vi "BMU参数读取-Auto.vi"(7 "Socket":dbl, 8 "CAN端口":u16(ring), 9 "设备索引号":u16(ring), 10 "CAN卡类型":u32(ring)=21, 11 "从板号":u8=1) -> (3 "成功?":bool)   [LabVIEW 2013] (continued)
      n13 = property on="电池额定容量(A)" class="DigNum (严格)"("Disabled"=w44) -> ()  [unwired: 2 in, 2 out]
      n14 = local write "主从选择"(enum32{"主板", "从板"}."从板" ("主从选择")) -> ()
      n15 = property on="SOC(%)" class="DigNum (严格)"("Disabled"=w44) -> ()  [unwired: 2 in, 2 out]
      n16 = local write "等级 2"(T20."从板信息" ("等级 2")) -> ()
      n17 = local write "主板2"(T9."项目信息" ("主从板")) -> ()
      n18 = property class="MCListbox (严格)"(reference=w49, "ItemNames"=w45) -> ()  [unwired: 1 in, 2 out]
      n19 = property class="MCListbox (严格)"(reference=w48, "ItemNames"=w45) -> ()  [unwired: 1 in, 2 out]
      n20 = property class="MCListbox (严格)"(reference=w47, "ItemNames"=w45) -> ()  [unwired: 1 in, 2 out]
      n21 = property class="Bool (严格)"(reference=w66, "BoolText.TextColor"=u32 87470) -> ()  [unwired: 1 in, 2 out]
      n22 = property class="Bool (严格)"(reference=w67, "BoolText.TextColor"=w41) -> ()  [unwired: 1 in, 2 out]
      n23 = property on="从板号" class="DigNum (严格)"("Visible"=TRUE ("可见")) -> ()  [unwired: 2 in, 2 out]
      n24 = local write "主从板"(enum32{"单选选项2", "单选选项1"}."单选选项1" ("主从板")) -> ()
      n25 = property on="项目信息2" class="Clust (严格)"("DisabledEnum"=w44) -> ()  [unwired: 2 in, 2 out]
      n26 = property on="系统时钟" class="Str"("Disabled"=w44) -> ()  [unwired: 2 in, 2 out]
      n27 = property on="配置文件版本" class="Str"("Disabled"=w44) -> ()  [unwired: 2 in, 2 out]
      n28 = property on="车架(牌)号" class="Str"("Disabled"=w44) -> ()  [unwired: 2 in, 2 out]
      n29 = property on="产品编号" class="Str"("Disabled"=w44) -> ()  [unwired: 2 in, 2 out]
      n30 = property on="单选选项2 2" class="Bool (严格)"("BoolText.TextColor"=w41) -> ()  [unwired: 2 in, 2 out]
      n31 = property on="单选选项2" class="Bool (严格)"("BoolText.TextColor"=w41) -> ()  [unwired: 2 in, 2 out]
      n32 = property on="单选选项1" class="Bool (严格)"("BoolText.TextColor"=u32 5898201) -> ()  [unwired: 2 in, 2 out]
      n33 = property on="从板号" class="DigNum (严格)"("NumText.BGColor"=w41) -> ()  [unwired: 2 in, 2 out]
      n34 = local write "面板选择"(T7."读写参数" ("面板选择")) -> ()
      n35 = local write "主界面选项"(enum32{"单选选项1", "单选选项2", "单选选项2 2", "单选选项2 3"}."单选选项1" ("主界面选项")) -> ()
      n36 = local write "判定3"(w51) -> ()
      n37 = local write "清BUFF"(w51) -> ()
      n38 = local write "1"(w51) -> ()
      n39 = property on="从板个数" class="DigNum (严格)"("Visible"=w51) -> ()  [unwired: 2 in, 2 out]
      n40 = property on="从板个数" class="DigNum (严格)"("NumText.BGColor"=u32 16448250) -> ()  [unwired: 2 in, 2 out]
      n41 = Not(x=w51) -> (.not. x?=w70:bool)
      n42 = property on="主板选项" class="Tree (严格)"("Visible"=w51) -> ()  [unwired: 2 in, 2 out]
      n43 = property on="全部写入" class="Bool (严格)"("DisabledEnum"=2) -> ()  [unwired: 2 in, 2 out]
      n44 = property on="当前从板板号" class="DigNum (严格)"("Visible"=w70) -> ()  [unwired: 2 in, 2 out]
      n45 = property on="从板选项" class="Tree (严格)"("Visible"=w70) -> ()  [unwired: 2 in, 2 out]
      n46 = control-ref of="结果"() -> (w57:refnum<vi>)
      n47 = control-ref of="结果"() -> (w54:refnum<vi>)
      n48 = local write "强制停止版本读取"(w43) -> ()
      n49 = local write "强制终止读写标记"(w43) -> ()
      n50 = control-ref of="项目信息"() -> (w55:refnum<vi>)
      n51 = local write "判定2"(w43) -> ()
      n52 = local write "停止"(w43) -> ()
      n53 = local write "控制1"(w43) -> ()
      n54 = local write "消除"(w43) -> ()
      n55 = global write "EV05全局变量1.vi" "授权功能"(w43) -> ()
      n56 = local write "继电器超时处理"(w43) -> ()
      n57 = local write "1 6"(w43) -> ()
      n58 = local write "1 7"(w43) -> ()
      n59 = local write "1 8"(w43) -> ()
      n60 = local write "1 9"(w43) -> ()
      n61 = local write "1 10"(w43) -> ()
      n62 = local write "1 2"(w43) -> ()
      n63 = local write "1 3"(w43) -> ()
      n64 = local write "1 4"(w43) -> ()
      n65 = local write "1 5"(w43) -> ()
      n66 = local write "1 11"(w43) -> ()
      n67 = for {
        N: 100 -> [_]
        tunnel: w57 -> [w98]
        i -> [w96]
        n68 = Bundle(w96, 0) -> (w94:cluster{i32, i32})  [unwired: 1 out]
        n69 = property class="MCListbox (严格)"(reference=w98, "ActiveCell"=w94, "CellBG"=u32 16448250) -> ()  [unwired: 1 in, 2 out]
      }
      n70 = for {
        N: 100 -> [_]
        tunnel: w55 -> [w93]
        i -> [w92]
        n71 = Bundle(w92, 0) -> (w90:cluster{i32, i32})  [unwired: 1 out]
        n72 = property class="Tbl (严格)"(reference=w93, "Active Cell"=w90, "Cell BG Color"=u32 16448250) -> ()  [unwired: 1 in, 2 out]
      }
      n73 = for {
        N: 100 -> [_]
        tunnel: w54 -> [w103]
        i -> [w101]
        n74 = Bundle(w101, 0) -> (w99:cluster{i32, i32})  [unwired: 1 out]
        n75 = property class="MCListbox (严格)"(reference=w103, "ActiveCell"=w99, "CellBG"=u32 16448250) -> ()  [unwired: 1 in, 2 out]
      }
      n76 = disable-structure shown="禁用" {
        disable-tunnel: [w71 _] -> w50
        frame Disabled {
          n77 = stacked-sequence {
            tunnel: [_ _ w77] -> w71
            frame #0 {
              w72 = u32 4 items=["PCI5121"=1, "PCI9810"=2, "USBCAN1"=3, "USBCAN2"=4, "PCI9820"=5, "PCI5110"=7, "CANLite(mini)"=8, "ISA9620"=9, "ISA5420"=10, "PC104CAN"=11, "DNP9810"=13, "PCI9840B"=14, "PC104C2"=15, "PCI9820I"=16, "pec9920"=18, "USBCAN_E_U"=20, "USBCAN_2E_U"=21] ("CAN卡类型")
              n78 = local write "CAN卡类型"(w72) -> ()
            }
            frame #1 {
              n79 = local read "设备索引号"() -> (w74:u16)
              n80 = local read "CAN卡类型"() -> (w73:u32)
              n81 = local read "CAN端口"() -> (w75:u16)
              n82 = dll-call lib="PTH1abs FBluewave New EnergySVN_WorkAutoTest_TestStandtrunkAutoTest_TestStandDriverZlgCanBHN01è¯»ååæ°data\nkerneldlls\nusbcan.dll" fn="VCI_ClearBuffer"("DeviceType"=w73, "DeviceInd"=w74, "CANInd"=w75) -> (error out=w76:errorcluster)  [unwired: 4 in, 4 out]
              n83 = call <vilib>:"Clear Errors.vi"("error in (no error)"=w76) -> ()  [unwired: 6 in, 1 out]
            }
            frame #2 {
              w84 = u8 0 items=["Normal", "Listen Only"] ("工作方式")
              w83 = u8 1 items=["Dual Filter", "Single Filter"] ("滤波方式")
              n84 = local read "CAN卡类型"() -> (w78:u32)
              n85 = local read "设备索引号"() -> (w79:u16)
              n86 = local read "CAN端口"() -> (w80:u16)
              n87 = call "CAN_Init-8.6.vi"("CAN卡类型"=w78, "设备索引号"=w79, "CAN端口"=w80, "操作类型"=enum16{"初始化CAN", "关闭CAN"}."初始化CAN", "滤波方式"=w83, "Accept Code"=u32 3221225472, "簇"=T22 {"打开CAN"=TRUE, "初始化CAN"=TRUE, "开始CAN"=TRUE, "重启"=FALSE, "关闭CAN"=FALSE}, "Mask Code"=u32 1073741823 ("Accept Code"), "工作方式"=w84, "是否滤波"=TRUE, "滤波选择"=T21 {"fiter_mode"=1, "fiter_endid"=402653184, "fiter_startid"=419430399}) -> ("error out"=w77:errorcluster)  [unwired: 3 in, 5 out]
            }
          }
        }
        frame Enabled {
        }
      }
      n88 = local write "加热继电器(从)"(w43) -> ()
      n89 = local write "风机继电器(从)"(w43) -> ()
      n90 = local write "DO1"(w43) -> ()
      n91 = local write "DO2"(w43) -> ()
      n92 = local write "DO1 2"(w43) -> ()
      n93 = local write "正级继电器"(w43) -> ()
      n94 = local write "负级继电器"(w43) -> ()
      n95 = local write "加热继电器"(w43) -> ()
      n96 = local write "充电继电器"(w43) -> ()
      n97 = local write "风机继电器"(w43) -> ()
      n98 = local write "预充电继电器"(w43) -> ()
      n99 = property on="保存版本信息" class="Bool (严格)"("Visible"=w43) -> ()  [unwired: 2 in, 2 out]
      n100 = property on="单个读取" class="Bool (严格)"("Visible"=w43) -> ()  [unwired: 2 in, 2 out]
      n101 = property on="单个写入" class="Bool (严格)"("Visible"=w43) -> ()  [unwired: 2 in, 2 out]
      n102 = local write "正级继电器 12"(w43) -> ()
      n103 = local write "正级继电器 2"(w43) -> ()
      n104 = local write "正级继电器 3"(w43) -> ()
      n105 = local write "正级继电器 4"(w43) -> ()
      n106 = local write "正级继电器 5"(w43) -> ()
      n107 = local write "正级继电器 6"(w43) -> ()
      n108 = local write "正级继电器 7"(w43) -> ()
      n109 = local write "正级继电器 8"(w43) -> ()
      n110 = local write "正级继电器 9"(w43) -> ()
      n111 = local write "正级继电器 10"(w43) -> ()
      n112 = local write "正级继电器 11"(w43) -> ()
      "电池故障" <- w45
      "模块版本值" <- w62
      "硬件版本" <- w63
      "模块版本名称" <- w62
      "平台软件版本" <- w63
      "项目软件版本" <- w63
      "模块个数" <- u8[] [0, 0, 0, 0, 0, 0, 0, 0, 0, 0, 0, 0, 0, 0, 0, 0, 0, 0, 0, 0, 0, 0, 0, 0, 0, 0, 0, 0, 0, 0, 0, 0] ("模块个数")
    }
  }
  n113 = stacked-sequence {
    tunnel: [w104] -> w29
    frame #0 {
      n114 = call <vilib>:"Set Busy.vi"() -> ()  [unwired: 10 in, 2 out]
      n115 = disable-structure shown="禁用" {
        frame Disabled {
          n116 = control-ref of="主板选项"() -> (w223:refnum<vi>)
          n117 = stacked-sequence {
            tunnel: w223 -> [w225 w383 w421]
            frame #0 {
              # "加热和充电控制参数"
              n118 = global read "功能码全局.vi" "主板控制类信息10"() -> (w235:bool[])
              n119 = Index Array(array=w235) -> (element #5=w229:bool, element #6=w227:bool, element #7=w228:bool, element #8=w226:bool)  [unwired: 8 in, 4 out]
              n120 = Not Or(1:w228, 2:w229) -> (0:w234:bool)
              n121 = Not Or(1:w226, 2:w227) -> (0:w232:bool)
              n122 = for {
                N: 8 -> [_]
                tunnel: w225 -> [w355]
                tunnel: w234 -> [w351]
                tunnel: [w350] -> w233
                i -> [w353]
                n123 = Add(x=w353, y=69) -> (x+y=w354:i32)
                n124 = property class="Tree (严格)"(reference=w355, "Active Item Row Number"=w354, "Disabled?"=w351) -> (error out=w350:errorcluster)  [unwired: 1 in, 1 out]
              }
              n125 = for {
                N: 9 -> [_]
                tunnel: w225 -> [w349]
                tunnel: w232 -> [w345]
                tunnel: w233 -> [w344]
                tunnel: [w343] -> w224
                i -> [w347]
                n126 = Add(x=w347, y=77) -> (x+y=w348:i32)
                n127 = property class="Tree (严格)"(reference=w349, error in=w344, "Active Item Row Number"=w348, "Disabled?"=w345) -> (error out=w343:errorcluster)  [unwired: 1 out]
              }
              n128 = stacked-sequence {
                tunnel: w225 -> [w255 _ _]
                tunnel: w224 -> [w254 _ _]
                frame #0 {
                  # "电池信息"
                  n129 = global read "功能码全局.vi" "主板版本号11"() -> (w256:bool[])
                  n130 = global read "功能码全局.vi" "主板项目信息4"() -> (w238:bool[])
                  n131 = Index Array(array=w256) -> (element #1=w252:bool, element #2=w251:bool, element #3=w245:bool, element #4=w239:bool, element #6=w244:bool, element #7=w243:bool, element #8=w242:bool)  [unwired: 8 in, 1 out]
                  n132 = Index Array(array=w238, index=4 ("索引")) -> (element=w236:bool)
                  n133 = Or(x=w245, y=w239) -> (x .or. y?=w240:bool)
                  n134 = Not(x=w243) -> (.not. x?=w247:bool)
                  n135 = Not(x=w242) -> (.not. x?=w246:bool)
                  n136 = Not(x=w244) -> (.not. x?=w248:bool)
                  n137 = property on="硬件版本号" class="Str"("Visible"=w245) -> ()  [unwired: 2 in, 2 out]
                  n138 = property on="读硬件版本号" class="Bool (严格)"("Visible"=w245) -> ()  [unwired: 2 in, 2 out]
                  n139 = property on="项目软件版本号" class="Str"("Visible"=w245) -> ()  [unwired: 2 in, 2 out]
                  n140 = property on="项目软本读取" class="Bool (严格)"("Visible"=w245) -> ()  [unwired: 2 in, 2 out]
                  n141 = property on="继电器屏1 2" class="TabCtl (严格)"("Visible"=w248) -> ()  [unwired: 2 in, 2 out]
                  n142 = property on="均衡屏" class="TabCtl (严格)"("Visible"=w246) -> ()  [unwired: 2 in, 2 out]
                  n143 = property on="继电器屏1 2" class="TabCtl (严格)"("Visible"=w248) -> ()  [unwired: 2 in, 2 out]
                  n144 = property on="DO屏" class="TabCtl (严格)"("Visible"=w247) -> ()  [unwired: 2 in, 2 out]
                  n145 = Compound Arithmetic op=OR(w244, w243, w242) -> (w241:bool)
                  n146 = Not Or(1:w251, 2:w252) -> (0:w250:bool)
                  n147 = stacked-sequence {
                    tunnel: w241 -> [_ w261 _]
                    tunnel: w240 -> [_ _ w265]
                    tunnel: w236 -> [w257 _ _]
                    frame #0 {
                      n148 = case shown="真" w257 {
                        frame False {
                        }
                        frame True {
                          n149 = local write "主界面选项"(enum32{"单选选项1", "单选选项2", "单选选项2 2", "单选选项2 3"}."单选选项2 3" ("主界面选项")) -> ()
                          n150 = local write "面板选择"(T7."高压板校正" ("面板选择")) -> ()
                        }
                      }
                      n151 = control-ref of="单选选项2 3"() -> (w258:refnum<vi>)
                      n152 = property class="Bool (严格)"(reference=w258, "Visible"=w257) -> ()  [unwired: 1 in, 2 out]
                    }
                    frame #1 {
                      n153 = control-ref of="单选选项2 2"() -> (w262:refnum<vi>)
                      n154 = case shown="真" w261 {
                        frame False {
                        }
                        frame True {
                          n155 = local write "主界面选项"(enum32{"单选选项1", "单选选项2", "单选选项2 2", "单选选项2 3"}."单选选项2 2" ("主界面选项")) -> ()
                          n156 = local write "面板选择"(enum32{"读写参数", "版本读取", "其它诊断"}."其它诊断" ("选项卡控件 2")) -> ()
                        }
                      }
                      n157 = property class="Bool (严格)"(reference=w262, "Visible"=w261) -> ()  [unwired: 1 in, 2 out]
                    }
                    frame #2 {
                      n158 = control-ref of="单选选项2"() -> (w266:refnum<vi>)
                      n159 = case shown="真" w265 {
                        frame False {
                        }
                        frame True {
                          n160 = local write "主界面选项"(enum32{"单选选项1", "单选选项2", "单选选项2 2", "单选选项2 3"}."单选选项2" ("主界面选项")) -> ()
                          n161 = local write "面板选择"(enum32{"读写参数", "版本读取", "其它诊断"}."版本读取" ("选项卡控件 2")) -> ()
                        }
                      }
                      n162 = property class="Bool (严格)"(reference=w266, "Visible"=w265) -> ()  [unwired: 1 in, 2 out]
                    }
                  }
                  n163 = for {
                    N: 5 -> [_]
                    tunnel: w255 -> [w275]
                    tunnel: w250 -> [w271]
                    tunnel: w254 -> [w270]
                    tunnel: [w269] -> w253
                    i -> [w273]
                    n164 = Add(x=w273, y=86) -> (x+y=w274:i32)
                    n165 = property class="Tree (严格)"(reference=w275, error in=w270, "Active Item Row Number"=w274, "Disabled?"=w271) -> (error out=w269:errorcluster)  [unwired: 1 out]
                  }
                  n166 = property on="模块软件版本 2" class="MCListbox (严格)"("Visible"=w239) -> ()  [unwired: 2 in, 2 out]
                  n167 = property on="模块软件版本" class="Enum (严格)"("Visible"=w239) -> ()  [unwired: 2 in, 2 out]
                  n168 = property on="平台软件版本号" class="Str"("Visible"=w239) -> ()  [unwired: 2 in, 2 out]
                  n169 = property on="模块版本读取" class="Bool (严格)"("Visible"=w239) -> ()  [unwired: 2 in, 2 out]
                  n170 = property on="平台软件版本读取" class="Bool (严格)"("Visible"=w239) -> ()  [unwired: 2 in, 2 out]
                  n171 = call <vilib>:"Clear Errors.vi"("error in (no error)"=w253) -> ()  [unwired: 6 in, 1 out]
                }
                frame #1 {
                  n172 = global read "功能码全局.vi" "主板项目信息7"() -> (w315:bool[])
                  n173 = global read "功能码全局.vi" "主板控制类信息10"() -> (w311:bool[])
                  n174 = global read "功能码全局.vi" "主板故障阀值9"() -> (w314:bool[])
                  n175 = global read "功能码全局.vi" "主板项目信息4"() -> (w293:bool[])
                  n176 = global read "功能码全局.vi" "主板项目信息5"() -> (w302:bool[])
                  n177 = global read "功能码全局.vi" "主板项目信息6"() -> (w292:bool[])
                  n178 = global read "功能码全局.vi" "主板版本号11"() -> (w301:bool[])
                  n179 = Delete From Array(array=w292, length=1 ("长度"), index=0 ("索引")) -> (deleted portion=w303:bool[], array with subset deleted=w319:bool[])
                  n180 = Index Array(array=w293, index #1=5 ("索引"), index #2=6 ("索引"), index #3=7 ("索引")) -> (element #1=w304:bool, element #2=w320:bool, element #3=w276:bool)
                  n181 = Index Array(array=w301) -> (element #1=w308:bool, element #2=w324:bool)  [unwired: 2 in]
                  n182 = Array Subset(array=w314, index=2 ("索引"), length=3 ("长度")) -> (w306:bool[])
                  n183 = Delete From Array(array=w315, length=3 ("索引"), index=2 ("长度")) -> (deleted portion=w305:bool[], array with subset deleted=w321:bool[])
                  n184 = Array Subset(array=w311, index=4 ("索引"), length=2 ("长度")) -> (w307:bool[])
                  n185 = global read "功能码全局.vi" "18"() -> (w284:bool[])
                  n186 = global read "功能码全局.vi" "16"() -> (w285:bool[])
                  n187 = Insert Into Array(array=w302, new element #1=w303, new element #2=w304, new element #3=w305, new element #4=w306, new element #5=w307, new element #6=w308) -> (w325:bool[])  [unwired: 1 in]
                  n188 = Array Subset(array=w311, index=6 ("索引"), length=2 ("长度")) -> (w323:bool[])
                  n189 = Array Subset(array=w314, index=5 ("索引"), length=3 ("长度")) -> (w322:bool[])
                  n190 = And Array Elements(Boolean array=w325) -> (logical AND=w290:bool)
                  n191 = Array Subset(array=w284, index=0 ("索引"), length=8 ("长度")) -> (w282:bool[])
                  n192 = Array Subset(array=w285, index=4 ("索引"), length=4 ("长度")) -> (w281:bool[])
                  n193 = Or Array Elements(Boolean array=w325) -> (logical OR=w277:bool)
                  n194 = Insert Into Array(array=w319, new element #1=w320, new element #2=w321, new element #3=w322, new element #4=w323, new element #5=w324) -> (w326:bool[])  [unwired: 1 in]
                  n195 = property on="全部读取" class="Bool (严格)"("Visible"=w290) -> ()  [unwired: 2 in, 2 out]
                  n196 = global read "功能码全局.vi" "15"() -> (w283:bool[])
                  n197 = And Array Elements(Boolean array=w326) -> (logical AND=w291:bool)
                  n198 = property on="全部写入" class="Bool (严格)"("Visible"=w291) -> ()  [unwired: 2 in, 2 out]
                  n199 = Or Array Elements(Boolean array=w326) -> (logical OR=w327:bool)
                  n200 = Insert Into Array(array=w283, new element #1=w282, new element #2=w281) -> (w280:bool[])  [unwired: 1 in]
                  n201 = Or Array Elements(Boolean array=w280) -> (logical OR=w279:bool)
                  n202 = Compound Arithmetic op=OR(w276, w277, w327, w279) -> (w328:bool)
                  n203 = case shown="真" w328 {
                    frame False {
                    }
                    frame True {
                      n204 = local write "主界面选项"(enum32{"单选选项1", "单选选项2", "单选选项2 2", "单选选项2 3"}."单选选项1" ("主界面选项")) -> ()
                      n205 = local write "面板选择"(enum32{"读写参数", "版本读取", "其它诊断"}."读写参数" ("选项卡控件 2")) -> ()
                    }
                  }
                  n206 = property on="单选选项1" class="Bool (严格)"("Visible"=w328) -> ()  [unwired: 2 in, 2 out]
                }
                frame #2 {
                  n207 = control-ref of="单选选项2 2"() -> (w335:refnum<vi>)
                  n208 = control-ref of="单选选项2 3"() -> (w331:refnum<vi>)
                  n209 = control-ref of="单选选项2"() -> (w337:refnum<vi>)
                  n210 = control-ref of="单选选项1"() -> (w336:refnum<vi>)
                  n211 = local read "主界面选项"() -> (w340:enum32{"单选选项1", "单选选项2", "单选选项2 2", "单选选项2 3"})
                  n212 = Build Array(w336, w337, w335, w331) -> (w334:refnum<vi>[])
                  n213 = Delete From Array(array=w334, index=w340) -> (deleted portion=w338:refnum<vi>, array with subset deleted=w339:refnum<vi>[])  [unwired: 1 in]
                  n214 = property class="Bool (严格)"(reference=w338, "BoolText.TextColor"=u32 87470) -> ()  [unwired: 1 in, 2 out]
                  n215 = for {
                    tunnel: u32 16777215 -> [w342]
                    tunnel: w339 -> [w341] mode=indexing
                    n216 = property class="Bool (严格)"(reference=w341, "BoolText.TextColor"=w342) -> ()  [unwired: 1 in, 2 out]
                  }
                }
              }
            }
            frame #1 {
              # "项目信息"
              # "SOC"
              # "SOH"
              # "电池额定实际容量"
              # "车牌号"
              # "产品编号"
              # "电压个数"
              # "通道电压数"
              # "温度个数"
              # "电压起始值"
              # "温度起始值"
              # "配置文件版本"
              # "系统时钟"
              # "校正时钟"
              n217 = global read "功能码全局.vi" "主板项目信息5"() -> (w416:bool[])
              n218 = global read "功能码全局.vi" "主板项目信息6"() -> (w415:bool[])
              n219 = global read "功能码全局.vi" "主板项目信息7"() -> (w392:bool[])
              n220 = global read "功能码全局.vi" "主板项目信息4"() -> (w363:bool[])
              n221 = Index Array(array=w416) -> (element #1=w413:bool, element #2=w410:bool, element #3=w407:bool, element #4=w404:bool, element #5=w400:bool, element #6=w398:bool, element #7=w395:bool, element #8=w391:bool)  [unwired: 8 in]
              n222 = Index Array(array=w415) -> (element #1=w388:bool, element #2=w412:bool, element #3=w409:bool, element #4=w406:bool, element #5=w403:bool, element #6=w399:bool, element #7=w397:bool, element #8=w394:bool)  [unwired: 8 in]
              n223 = Index Array(array=w392) -> (element #1=w390:bool, element #2=w387:bool, element #3=w385:bool, element #4=w380:bool, element #5=w377:bool, element #6=w384:bool, element #7=w378:bool, element #8=w376:bool)  [unwired: 8 in]
              n224 = Index Array(array=w363) -> (element #6=w359:bool, element #7=w358:bool, element #8=w362:bool)  [unwired: 8 in, 5 out]
              n225 = Not(x=w362) -> (.not. x?=w361:bool)
              n226 = Not Or(1:w358, 2:w359) -> (0:w357:bool)
              n227 = Not Or(1:w412, 2:w413) -> (0:w375:bool)
              n228 = Not Or(1:w409, 2:w410) -> (0:w374:bool)
              n229 = Not Or(1:w406, 2:w407) -> (0:w373:bool)
              n230 = Not Or(1:w403, 2:w404) -> (0:w372:bool)
              n231 = Not Or(1:w399, 2:w400) -> (0:w371:bool)
              n232 = Not Or(1:w397, 2:w398) -> (0:w370:bool)
              n233 = Not Or(1:w394, 2:w395) -> (0:w369:bool)
              n234 = Not Or(1:w390, 2:w391) -> (0:w368:bool)
              n235 = Not Or(1:w384, 2:w385) -> (0:w366:bool)
              n236 = Not Or(1:w376, 2:w377) -> (0:w364:bool)
              n237 = Not Or(1:w378, 2:w380) -> (0:w365:bool)
              n238 = Not Or(1:w387, 2:w388) -> (0:w367:bool)
              n239 = Compound Arithmetic op=OR(w361, w375, w374, w373, w372, w371, w370, w369, w368, w367, w366, w365, w364) -> (w356:bool)
              "项目信息结果" <- w356
              n240 = property class="Tree (严格)"(reference=w383, "Active Item Row Number"=9 ("活动项:行数"), "Disabled?"=w357, "Active Item Row Number"=1 ("活动项:行数"), "Disabled?"=w356, "Active Item Row Number"=0 ("活动项:行数"), "Disabled?"=w361, "Active Item Row Number"=3 ("活动项:行数"), "Disabled?"=w375, "Active Item Row Number"=4 ("活动项:行数"), "Disabled?"=w374, "Active Item Row Number"=5 ("活动项:行数"), "Disabled?"=w373, "Active Item Row Number"=6 ("活动项:行数"), "Disabled?"=w372, "Active Item Row Number"=7 ("活动项:行数"), "Disabled?"=w371, "Active Item Row Number"=8 ("活动项:行数"), "Disabled?"=w370, "Active Item Row Number"=11 ("活动项:行数"), "Disabled?"=w369, "Active Item Row Number"=12 ("活动项:行数"), "Disabled?"=w368, "Active Item Row Number"=13 ("活动项:行数"), "Disabled?"=w367, "Active Item Row Number"=2 ("活动项:行数"), "Disabled?"=w366, "Active Item Row Number"=10 ("活动项:行数"), "Disabled?"=w365, "Active Item Row Number"=14 ("活动项:行数"), "Disabled?"=w364) -> ()  [unwired: 1 in, 2 out]
            }
            frame #2 {
              w426 = 18
              # "一二三级故障"
              n241 = global read "功能码全局.vi" "主板故障阀值9"() -> (w432:bool[])
              n242 = Index Array(array=w432) -> (element #3=w431:bool, element #4=w428:bool, element #5=w425:bool, element #6=w430:bool, element #7=w427:bool, element #8=w424:bool)  [unwired: 8 in, 2 out]
              n243 = Not Or(1:w430, 2:w431) -> (0:w420:bool)
              n244 = Not Or(1:w427, 2:w428) -> (0:w418:bool)
              n245 = Not Or(1:w424, 2:w425) -> (0:w419:bool)
              n246 = for {
                N: w426 -> [_]
                tunnel: w421 -> [w452]
                tunnel: w420 -> [w448]
                tunnel: [w447] -> w429
                i -> [w450]
                n247 = Add(x=w450, y=15) -> (x+y=w451:i32)
                n248 = property class="Tree (严格)"(reference=w452, "Active Item Row Number"=w451, "Disabled?"=w448) -> (error out=w447:errorcluster)  [unwired: 1 in, 1 out]
              }
              n249 = for {
                N: w426 -> [_]
                tunnel: w421 -> [w446]
                tunnel: w418 -> [w442]
                tunnel: w429 -> [w441]
                tunnel: [w440] -> w423
                i -> [w444]
                n250 = Add(x=w444, y=33) -> (x+y=w445:i32)
                n251 = property class="Tree (严格)"(reference=w446, error in=w441, "Active Item Row Number"=w445, "Disabled?"=w442) -> (error out=w440:errorcluster)  [unwired: 1 out]
              }
              n252 = for {
                N: w426 -> [_]
                tunnel: w421 -> [w439]
                tunnel: w419 -> [w435]
                tunnel: w423 -> [w434]
                tunnel: [w433] -> w422
                i -> [w437]
                n253 = Add(x=w437, y=51) -> (x+y=w438:i32)
                n254 = property class="Tree (严格)"(reference=w439, error in=w434, "Active Item Row Number"=w438, "Disabled?"=w435) -> (error out=w433:errorcluster)  [unwired: 1 out]
              }
              n255 = call <vilib>:"Clear Errors.vi"("error in (no error)"=w422) -> ()  [unwired: 6 in, 1 out]
            }
          }
        }
        frame Enabled {
        }
      }
      n256 = disable-structure shown="禁用" {
        disable-tunnel: [w105 _] -> w104
        frame Disabled {
          n257 = control-ref of="从板选项"() -> (w106:refnum<vi>)
          n258 = stacked-sequence {
            tunnel: w106 -> [w109 w146 w188]
            tunnel: [w107 _ _] -> w105
            frame #0 {
              n259 = global read "功能码全局.vi" "15"() -> (w132:bool[])
              n260 = global read "功能码全局.vi" "16"() -> (w123:bool[])
              n261 = Index Array(array=w132) -> (element #1=w131:bool, element #2=w129:bool, element #3=w127:bool, element #4=w125:bool, element #5=w130:bool, element #6=w128:bool, element #7=w126:bool, element #8=w124:bool)  [unwired: 8 in]
              n262 = Index Array(array=w123) -> (element #5=w114:bool, element #6=w122:bool, element #7=w113:bool, element #8=w121:bool)  [unwired: 8 in, 4 out]
              n263 = Not Or(1:w121, 2:w122) -> (0:w111:bool)
              n264 = Not Or(1:w113, 2:w114) -> (0:w112:bool)
              n265 = Not Or(1:w130, 2:w131) -> (0:w117:bool)
              n266 = Not Or(1:w128, 2:w129) -> (0:w118:bool)
              n267 = Not Or(1:w126, 2:w127) -> (0:w119:bool)
              n268 = Not Or(1:w124, 2:w125) -> (0:w120:bool)
              n269 = Compound Arithmetic op=OR(w117, w118, w119, w120, w111) -> (w116:bool)
              "从板项目信息" <- w116
              n270 = property class="Tree (严格)"(reference=w109, "Active Item Row Number"=1 ("活动项:行数"), "Disabled?"=w116, "Active Item Row Number"=2 ("活动项:行数"), "Disabled?"=w117, "Active Item Row Number"=3 ("活动项:行数"), "Disabled?"=w118, "Active Item Row Number"=4 ("活动项:行数"), "Disabled?"=w119, "Active Item Row Number"=5 ("活动项:行数"), "Disabled?"=w120, "Active Item Row Number"=0 ("活动项:行数"), "Disabled?"=w112) -> (error out=w108:errorcluster)  [unwired: 1 in, 1 out]
              n271 = for {
                N: 8 -> [_]
                tunnel: w109 -> [w144]
                tunnel: w111 -> [w140]
                tunnel: w108 -> [w139]
                tunnel: [w138] -> w107
                i -> [w142]
                n272 = Add(x=w142, y=6) -> (x+y=w143:i32)
                n273 = property class="Tree (严格)"(reference=w144, error in=w139, "Active Item Row Number"=w143, "Disabled?"=w140) -> (error out=w138:errorcluster)  [unwired: 1 out]
              }
              n274 = call <vilib>:"Clear Errors.vi"("error in (no error)"=w107) -> ()  [unwired: 6 in, 1 out]
            }
            frame #1 {
              w157 = 8
              n275 = global read "功能码全局.vi" "18"() -> (w166:bool[])
              n276 = Index Array(array=w166) -> (element #1=w149:bool, element #2=w150:bool, element #3=w165:bool, element #4=w160:bool, element #5=w154:bool, element #6=w164:bool, element #7=w159:bool, element #8=w153:bool)  [unwired: 8 in]
              n277 = Not Or(1:w150, 2:w149) -> (0:w145:bool)
              n278 = property class="Tree (严格)"(reference=w146, "Active Item Row Number"=46 ("活动项:行数"), "Disabled?"=w145, "Active Item Row Number"=47 ("活动项:行数"), "Disabled?"=w145, "Active Item Row Number"=48 ("活动项:行数"), "Disabled?"=w145) -> ()  [unwired: 1 in, 2 out]
              n279 = Not Or(1:w153, 2:w154) -> (0:w152:bool)
              n280 = Not Or(1:w164, 2:w165) -> (0:w163:bool)
              n281 = Not Or(1:w159, 2:w160) -> (0:w158:bool)
              n282 = for {
                N: w157 -> [_]
                tunnel: w146 -> [w187]
                tunnel: w163 -> [w183]
                tunnel: "error out" -> [w182]
                tunnel: [w181] -> w161
                i -> [w185]
                n283 = Add(x=w185, y=14) -> (x+y=w186:i32)
                n284 = property class="Tree (严格)"(reference=w187, error in=w182, "Active Item Row Number"=w186, "Disabled?"=w183) -> (error out=w181:errorcluster)  [unwired: 1 out]
              }
              n285 = for {
                N: w157 -> [_]
                tunnel: w146 -> [w180]
                tunnel: w158 -> [w176]
                tunnel: w161 -> [w175]
                tunnel: [w174] -> w156
                i -> [w178]
                n286 = Add(x=w178, y=22) -> (x+y=w179:i32)
                n287 = property class="Tree (严格)"(reference=w180, error in=w175, "Active Item Row Number"=w179, "Disabled?"=w176) -> (error out=w174:errorcluster)  [unwired: 1 out]
              }
              n288 = for {
                N: w157 -> [_]
                tunnel: w146 -> [w173]
                tunnel: w152 -> [w169]
                tunnel: w156 -> [w168]
                tunnel: [w167] -> w155
                i -> [w171]
                n289 = Add(x=w171, y=30) -> (x+y=w172:i32)
                n290 = property class="Tree (严格)"(reference=w173, error in=w168, "Active Item Row Number"=w172, "Disabled?"=w169) -> (error out=w167:errorcluster)  [unwired: 1 out]
              }
              n291 = call <vilib>:"Clear Errors.vi"("error in (no error)"=w155) -> ()  [unwired: 6 in, 1 out]
            }
            frame #2 {
              n292 = global read "功能码全局.vi" "23"() -> (w212:bool[])
              n293 = global read "功能码全局.vi" "24"() -> (w210:bool[])
              n294 = Index Array(array=w212) -> (element #3=w211:bool, element #4=w208:bool, element #5=w206:bool, element #6=w204:bool, element #7=w202:bool, element #8=w200:bool)  [unwired: 8 in, 2 out]
              n295 = Index Array(array=w210) -> (element #3=w209:bool, element #4=w207:bool, element #5=w205:bool, element #6=w203:bool, element #7=w201:bool, element #8=w199:bool)  [unwired: 8 in, 2 out]
              n296 = Not Or(1:w209, 2:w211) -> (0:w198:bool)
              n297 = Not Or(1:w207, 2:w208) -> (0:w193:bool)
              n298 = Not Or(1:w205, 2:w206) -> (0:w194:bool)
              n299 = Not Or(1:w203, 2:w204) -> (0:w195:bool)
              n300 = Not Or(1:w201, 2:w202) -> (0:w197:bool)
              n301 = Not Or(1:w199, 2:w200) -> (0:w196:bool)
              n302 = Build Array(w198, w198, w197, w196, w195, w194, w193) -> (w191:bool[])
              n303 = And Array Elements(Boolean array=w191) -> (logical AND=w192:bool)
              n304 = Insert Into Array(array=w191, index=0 ("索引"), new element=w192) -> (w189:bool[])
              n305 = for {
                N: 8 -> [_]
                tunnel: w188 -> [w222]
                tunnel: w189 -> [w218] mode=indexing
                tunnel: errorcluster {"status"=FALSE, "code"=0, "source"=""} ("error out 2") -> [w217]
                tunnel: [w216] -> w214
                i -> [w220]
                n306 = Add(x=w220, y=38) -> (x+y=w221:i32)
                n307 = property class="Tree (严格)"(reference=w222, error in=w217, "Active Item Row Number"=w221, "Disabled?"=w218) -> (error out=w216:errorcluster)  [unwired: 1 out]
              }
              n308 = call <vilib>:"Clear Errors.vi"("error in (no error)"=w214) -> ()  [unwired: 6 in, 1 out]
            }
          }
        }
        frame Enabled {
        }
      }
    }
  }
  n309 = Index Array(array=w19, index (col)=0 ("索引 (行)")) -> (element=w22:string[])  [unwired: 1 in]
  n310 = Index Array(array=w19, index (col)=1 ("禁用的索引 (列)")) -> (element=w12:string[])  [unwired: 1 in]
  n311 = local read "从板个数"() -> (w14:dbl)
  n312 = Array Subset(array=w22, index=0 ("索引"), length=w14) -> (w21:string[])
  n313 = Array Subset(array=w22, index=10 ("索引"), length=w14) -> (w20:string[])
  n314 = Array Subset(array=w12, index=0 ("索引"), length=w14) -> (w18:string[])
  n315 = Array Subset(array=w12, index=10 ("索引"), length=w14) -> (w13:string[])
  n316 = Insert Into Array(array=w21, new element=w20) -> (w11:string[])  [unwired: 1 in]
  n317 = Insert Into Array(array=w18, new element=w13) -> (w10:string[])  [unwired: 1 in]
  n318 = Build Array(w11, w10) -> (w9:string[][])
  n319 = local write "停止"(FALSE ("停止")) -> ()
  n320 = local write "项目信息 2"(string[][] [["电压个数", "36"], ["温度个数", "45"], ["第一个保险通道", "0"], ["第一个保险位置", "0"], ["第二个保险通道", "0"], ["第二个保险位置", "0"], ["第三个保险通道", "0"], ["第三个保险位置", "0"], ["第四个保险通道", "0"], ["第四个保险位置", "0"], ["第五个保险通道", "0"], ["第五个保险位置", "0"], ["第六个保险通道", "0"], ["第六个保险位置", "0"], ["第七个保险通道", "0"], ["第七个保险位置", "0"], ["第八个保险通道", "0"], ["第八个保险位置", "0"], ["第九个保险通道", "0"], ["第九个保险位置", "0"], ["第十个保险通道", "0"], ["第十个保险位置", "0"], ["第1通道电压个数", "11"], ["第2通道电压个数", "12"], ["第3通道电压个数", "12"], ["第4通道电压个数", "12"], ["第5通道电压个数", "12"]] ("项目信息 2")) -> ()
  n321 = Transpose 2D Array(2D array=w9) -> (transposed array=w8:string[][])
  n322 = local write "项目信息"(w8) -> ()
  n323 = stacked-sequence {
    tunnel: w26 -> [_]
    tunnel: w29 -> [_]
    frame #0 {
      n324 = call <vilib>:"Unset Busy.vi"() -> ()  [unwired: 11 in, 1 out]
    }
  }
  n325 = disable-structure shown="启用" {
    disable-tunnel: [w455 _] -> w37
    disable-tunnel: w26 -> [w454 w457]
    disable-tunnel: [w453 w457] -> w6
    frame Disabled {
      w456 = "CMD" ("名称（未命名）")
      n326 = Obtain Queue(name (unnamed)=w456, element data type=w456, error in (no error)=w454) -> (queue out=w455:refnum<queue>, error out=w453:errorcluster)  [unwired: 2 in, 1 out]
    }
    frame Enabled {
    }
  }
  n327 = Number To Decimal String(number="Socket") -> (decimal integer string=w2:string)  [unwired: 1 in]
  n328 = Concatenate Strings("Recv" ("字符串"), w2) -> (w1:string)
  n329 = Obtain Queue(name (unnamed)=w1, element data type="读参数") -> (queue out=w31:refnum<queue>, error out=w30:errorcluster)  [unwired: 3 in, 1 out]
  n330 = case shown="无错误" w6 {
    selector: w6 -> [w458 _]
    frame No Error {
      n331 = case shown="\"全部读取\"" "全部读取" {
        tunnel: w458 -> [_ _ _ _ w1099 _ _ _ _ _ _ _ _ _ _]
        frame "假", Default {
          n332 = local write "强制终止读写标记"(FALSE ("强制终止读写标记")) -> ()
        }
        frame "单个写入" {
          n333 = local read "主从选择"() -> (w469:enum32{"主板", "从板"})
          n334 = case shown="\"从板\"" w469 {
            tunnel: [w480 w495] -> w466
            tunnel: [0.0 w493] -> w470
            tunnel: [_ w494] -> w468
            tunnel: [w478 _] -> w467
            frame "主板", Default {
              n335 = flat-sequence {
                tunnel: [w492] -> w478
                frame #0 {
                  n336 = control-ref of="高压参数"() -> (w483:refnum<vi>)
                  n337 = control-ref of="电池信息"() -> (w484:refnum<vi>)
                  n338 = control-ref of="一级故障"() -> (w490:refnum<vi>)
                  n339 = control-ref of="一级故障 2"() -> (w488:refnum<vi>)
                  n340 = control-ref of="一级故障 3"() -> (w487:refnum<vi>)
                  n341 = control-ref of="加热控制参数"() -> (w486:refnum<vi>)
                  n342 = control-ref of="充电控制参数"() -> (w485:refnum<vi>)
                  n343 = control-ref of="项目信息"() -> (w489:refnum<vi>)
                  n344 = control-ref of="项目信息2"() -> (w491:refnum<vi>)
                  n345 = local read "主板数据"() -> (w481:T4)
                  n346 = Bundle(cluster=w481, "项目信息"=w489, "一级故障 4"=w491, "一级故障"=w490, "一级故障 2"=w488, "一级故障 3"=w487, "加热控制参数"=w486, "充电控制参数"=w485, "高压参数"=w483, "电池信息"=w484) -> (w482:T4)
                  n347 = local write "主板数据"(w482) -> ()
                }
                frame #1 {
                  n348 = control-ref of="主板数据"() -> (w492:refnum<vi>)
                }
              }
              n349 = local read "主板选项"() -> (w480:string)
            }
            frame "从板" {
              n350 = stacked-sequence {
                tunnel: [_ w506] -> w494
                frame #0 {
                  n351 = control-ref of="从板号"() -> (w505:refnum<vi>)
                  n352 = control-ref of="项目信息 2"() -> (w504:refnum<vi>)
                  n353 = control-ref of="均衡参数"() -> (w499:refnum<vi>)
                  n354 = control-ref of="加热控制参数"() -> (w503:refnum<vi>)
                  n355 = control-ref of="一级故障(从板)"() -> (w502:refnum<vi>)
                  n356 = control-ref of="二级故障(从板)"() -> (w501:refnum<vi>)
                  n357 = control-ref of="三级故障(从板)"() -> (w500:refnum<vi>)
                  n358 = control-ref of="电池组信息"() -> (w496:refnum<vi>)
                  n359 = local read "从板信息"() -> (w497:T2)
                  n360 = Bundle(cluster=w497, "从板号"=w505, "项目信息 2"=w504, "加热控制参数"=w503, "一级故障(从板)"=w502, "二级故障(从板)"=w501, "三级故障(从板)"=w500, "电池组信息(从板)"=w496, "均衡参数"=w499) -> (w498:T2)
                  n361 = local write "从板信息"(w498) -> ()
                }
                frame #1 {
                  n362 = control-ref of="从板信息"() -> (w506:refnum<vi>)
                }
              }
              n363 = local read "从板选项"() -> (w495:string)
              n364 = local read "从板号"() -> (w493:u8)
            }
          }
          n365 = local read "从板个数"() -> (w471:dbl)
          n366 = local read "二维码信息 2"() -> (w461:string)
          n367 = local read "二维码信息"() -> (w462:string)
          n368 = local read "快换"() -> (w472:bool)
          n369 = call "输入数据解析.vi"("单个参数补充"=w471, "从板号"=w470, "主板二维码"=w462, "从板二维码"=w461, "主板引用"=w467, "从板引用"=w468, "主板选项"=w466, "枚举"=w469, "快换"=w472) -> ("输出数组"=w476:dbl[][], "数组长度"=w475:dbl[], "循环次数"=w465:i32, "命令"=w474:u32, "名称"=w464:string[], "命令序号"=w473:u32[])  [unwired: 1 out]
          n370 = for {
            N: w465 -> [w512]
            tunnel: w476 -> [w522]
            tunnel: w475 -> [w521]
            tunnel: w474 -> [w520]
            tunnel: w473 -> [w519]
            tunnel: w470 -> [w510]
            tunnel: w466 -> [w518]
            tunnel: w464 -> [w514]
            tunnel: [w507] -> w463
            i -> [w513]
            n371 = Index Array(array=w522, index (row)=w513) -> (element=w517:dbl[])  [unwired: 1 in]
            n372 = Index Array(array=w521, index=w513) -> (element=w516:dbl)
            n373 = Index Array(array=w514, index=w513) -> (element=w511:string)
            n374 = case shown="\"假\", 默认" w511 {
              tunnel: [w524 w525] -> w509
              tunnel: w510 -> [w524 _]
              tunnel: [TRUE ("确定") w526] -> w508
              frame "假", Default {
              }
              frame "从板号" {
                n375 = call "请输入当前从板板号"() -> ("当前从板板号"=w525:dbl, "确定"=w526:bool)  [unwired: 17 in, 1 out]
                n376 = local write "当前从板板号"(w525) -> ()
              }
            }
            n377 = Index Array(array=w519, index=w513) -> (element=w515:u32)
            n378 = global write "全局 1.vi" "名称"(w511) -> ()
            n379 = case shown="真" w508 {
              tunnel: w520 -> [_ w536]
              tunnel: w518 -> [_ w535]
              tunnel: w517 -> [_ w534]
              tunnel: w516 -> [_ w533]
              tunnel: w515 -> [_ w532]
              tunnel: w513 -> [_ w531]
              tunnel: w511 -> [_ w530]
              tunnel: w512 -> [_ w529]
              tunnel: w509 -> [_ w528]
              tunnel: [_ w527] -> w507
              frame False {
                n380 = call <vilib>:"Unset Busy.vi"() -> ()  [unwired: 11 in, 1 out]
              }
              frame True {
                n381 = stacked-sequence {
                  seq-local: [_ _ _ w564 _ _] -> [_ _ _ _ w573 _]
                  tunnel: w534 -> [_ _ w549 _ _ _]
                  tunnel: w533 -> [_ _ w548 _ _ _]
                  tunnel: w536 -> [_ _ w542 _ _ _]
                  tunnel: w532 -> [_ _ w540 _ _ _]
                  tunnel: w535 -> [_ _ _ _ _ _]
                  tunnel: w531 -> [_ _ _ _ _ w584]
                  tunnel: w530 -> [_ _ _ _ w572 _]
                  tunnel: w529 -> [_ _ _ _ _ w585]
                  tunnel: w528 -> [_ _ w541 _ _ _]
                  tunnel: [_ _ _ _ _ w582] -> w527
                  frame #0 {
                    w538 = FALSE ("流控帧")
                    w537 = TRUE ("流控帧 2")
                    n382 = call <vilib>:"Set Busy.vi"("disable click? (T)"=w538) -> ()  [unwired: 3 in, 8 out]
                    n383 = global write "EV05全局变量1.vi" "读取超时"(w538) -> ()
                    n384 = global write "EV05全局变量1.vi" "流控帧"(w538) -> ()
                    n385 = local write "消除"(w537) -> ()
                    n386 = local write "控制1"(w537) -> ()
                    n387 = global write "EV05全局变量1.vi" "流控帧 2"(w537) -> ()
                    n388 = local write "写?"(w537) -> ()
                  }
                  frame #1 {
                    n389 = Wait Until Next ms Multiple(millisecond multiple=u32 50 ("毫秒倍数")) -> ()  [unwired: 1 out]
                  }
                  frame #2 {
                    n390 = local read "设备索引号"() -> (w544:u16)
                    n391 = local read "CAN卡类型"() -> (w545:u32)
                    n392 = Increment(x=w548) -> (x+1=w547:dbl)
                    n393 = local read "CAN端口"() -> (w543:u16)
                    n394 = local write "命令"(w542) -> ()
                    n395 = local write "命令序号"(w540) -> ()
                    n396 = Reshape Array(w549, w547) -> (w546:dbl[])
                    n397 = stacked-sequence {
                      tunnel: w546 -> [_ w563]
                      tunnel: w545 -> [w552 w562]
                      tunnel: w544 -> [w551 w561]
                      tunnel: w543 -> [w550 w560]
                      tunnel: w542 -> [_ w559]
                      tunnel: w541 -> [_ w558]
                      tunnel: w540 -> [_ w557]
                      frame #0 {
                        n398 = disable-structure shown="禁用" {
                          disable-tunnel: w552 -> [w555 _]
                          disable-tunnel: w551 -> [w554 _]
                          disable-tunnel: w550 -> [w553 _]
                          frame Disabled {
                            n399 = dll-call lib="PTH1abs FBluewave New EnergySVN_WorkAutoTest_TestStandtrunkAutoTest_TestStandDriverZlgCanBHN01è¯»ååæ°data\nkerneldlls\nusbcan.dll" fn="VCI_ClearBuffer"("DeviceType"=w555, "DeviceInd"=w554, "CANInd"=w553) -> (error out=w556:errorcluster)  [unwired: 4 in, 4 out]
                            n400 = call <vilib>:"Clear Errors.vi"("error in (no error)"=w556) -> ()  [unwired: 6 in, 1 out]
                          }
                          frame Enabled {
                          }
                        }
                      }
                      frame #1 {
                        n401 = call "多帧发送机制(EV05).vi"("can卡类型"=w562, "设备索引号"=w561, "CAN端口"=w560, "命令"=w559, "板号"=w558, "命令序号"=w557, "输入数据"=w563) -> ()  [unwired: 2 in, 11 out]
                      }
                    }
                  }
                  frame #3 {
                    n402 = while {
                      tunnel: [w566] -> w564
                      i -> [w570]
                      stop <- w567 stop-if-true
                      n403 = local read "强制终止读写标记"() -> (w565:bool)
                      n404 = global read "EV05全局变量1.vi" "读取超时"() -> (w566:bool)
                      n405 = Greater Or Equal?(x=w570, y=30) -> (x >= y?=w568:bool)
                      n406 = Wait Until Next ms Multiple(millisecond multiple=u32 100 ("毫秒倍数")) -> ()  [unwired: 1 out]
                      n407 = Compound Arithmetic op=OR(w565, w566, w568) -> (w567:bool)
                    }
                  }
                  frame #4 {
                    n408 = case shown="假" w573 {
                      tunnel: w572 -> [w574 w580]
                      frame False {
                        n409 = control-ref of="结果"() -> (w578:refnum<vi>)
                        n410 = Concatenate Strings(w574, "       写入失败" ("字符串")) -> (w577:string)
                        n411 = Build Array(w577) -> (w576:string[])
                        n412 = call "表格编辑.vi"("新元素/子数组"=w576, "活动单元格:单元格背景色"=u32 16740749, "MCListbox引用句柄"=w578) -> ()  [unwired: 9 out]
                      }
                      frame True {
                        n413 = case shown="\"从板号\"" w580 {
                          frame "假", Default {
                          }
                          frame "从板号" {
                            n414 = local read "从板号"() -> (w581:u8)
                            n415 = local write "当前从板板号"(w581) -> ()
                          }
                        }
                      }
                    }
                    n416 = call <vilib>:"Unset Busy.vi"() -> ()  [unwired: 2 in, 10 out]
                  }
                  frame #5 {
                    n417 = Increment(x=w584) -> (x+1=w583:i32)
                    n418 = Equal?(x=w585, y=w583) -> (x = y?=w582:bool)
                    n419 = case shown="真" w582 {
                      frame False {
                      }
                      frame True {
                        n420 = control-ref of="结果"() -> (w589:refnum<vi>)
                        n421 = Concatenate Strings("写入完成" ("字符串")) -> (w588:string)
                        n422 = Build Array(w588) -> (w587:string[])
                        n423 = call "表格编辑.vi"("新元素/子数组"=w587, "活动单元格:单元格背景色"=u32 21937, "MCListbox引用句柄"=w589) -> ()  [unwired: 9 out]
                      }
                    }
                  }
                }
              }
            }
          }
          n424 = stacked-sequence {
            tunnel: w463 -> [_]
            frame #0 {
              n425 = call <vilib>:"Unset Busy.vi"() -> ()  [unwired: 2 in, 10 out]
              n426 = local write "强制终止读写标记"(FALSE ("强制停止")) -> ()
            }
          }
        }
        frame "全部写入" {
          n427 = local read "主从选择"() -> (w596:enum32{"主板", "从板"})
          n428 = case shown="\"主板\", 默认" w596 {
            tunnel: [string[] ["项目信息", "一级故障阀值", "二级故障阀值", "三级故障阀值", "加热控制参数", "充电控制参数", "电池信息"] string[] ["从板信息", "一级故障阀值", "二级故障阀值", "三级故障阀值", "均衡参数"]] -> w593
            tunnel: [0.0 ("从板号") w725] -> w597
            tunnel: [w710 _] -> w595
            tunnel: [_ w726] -> w594
            frame "主板", Default {
              n429 = stacked-sequence {
                tunnel: [_ w724] -> w710
                frame #0 {
                  n430 = control-ref of="电池信息"() -> (w716:refnum<vi>)
                  n431 = control-ref of="高压参数"() -> (w715:refnum<vi>)
                  n432 = control-ref of="一级故障"() -> (w718:refnum<vi>)
                  n433 = control-ref of="一级故障 2"() -> (w720:refnum<vi>)
                  n434 = control-ref of="一级故障 3"() -> (w721:refnum<vi>)
                  n435 = control-ref of="加热控制参数"() -> (w722:refnum<vi>)
                  n436 = control-ref of="充电控制参数"() -> (w723:refnum<vi>)
                  n437 = control-ref of="项目信息"() -> (w719:refnum<vi>)
                  n438 = control-ref of="项目信息2"() -> (w717:refnum<vi>)
                  n439 = local read "主板数据"() -> (w714:T4)
                  n440 = Bundle(cluster=w714, "项目信息"=w719, "一级故障 4"=w717, "一级故障"=w718, "一级故障 2"=w720, "一级故障 3"=w721, "加热控制参数"=w722, "充电控制参数"=w723, "高压参数"=w715, "电池信息"=w716) -> (w713:T4)
                  n441 = local write "主板数据"(w713) -> ()
                }
                frame #1 {
                  n442 = control-ref of="主板数据"() -> (w724:refnum<vi>)
                }
              }
            }
            frame "从板" {
              (unwired) "均衡参数"
              n443 = stacked-sequence {
                tunnel: [_ w738] -> w726
                frame #0 {
                  n444 = control-ref of="从板号"() -> (w732:refnum<vi>)
                  n445 = control-ref of="项目信息 2"() -> (w733:refnum<vi>)
                  n446 = control-ref of="均衡参数"() -> (w730:refnum<vi>)
                  n447 = control-ref of="加热控制参数"() -> (w734:refnum<vi>)
                  n448 = control-ref of="一级故障(从板)"() -> (w735:refnum<vi>)
                  n449 = control-ref of="二级故障(从板)"() -> (w736:refnum<vi>)
                  n450 = control-ref of="三级故障(从板)"() -> (w737:refnum<vi>)
                  n451 = control-ref of="电池组信息"() -> (w731:refnum<vi>)
                  n452 = local read "从板信息"() -> (w729:T2)
                  n453 = Bundle(cluster=w729, "从板号"=w732, "项目信息 2"=w733, "加热控制参数"=w734, "一级故障(从板)"=w735, "二级故障(从板)"=w736, "三级故障(从板)"=w737, "电池组信息(从板)"=w731, "均衡参数"=w730) -> (w728:T2)
                  n454 = local write "从板信息"(w728) -> ()
                }
                frame #1 {
                  n455 = control-ref of="从板信息"() -> (w738:refnum<vi>)
                }
              }
              n456 = local read "从板号"() -> (w725:u8)
            }
          }
          n457 = Array Size(array=w593) -> (size(s)=w592:i32)
          n458 = while {
            tunnel: w593 -> [w605] mode=indexing
            tunnel: w596 -> [w609]
            tunnel: w597 -> [w612]
            tunnel: w595 -> [w611]
            tunnel: w594 -> [w610]
            tunnel: w592 -> [w603]
            tunnel: [w599] -> w591
            i -> [w604]
            stop <- w600 stop-if-true
            n459 = Increment(x=w604) -> (x+1=w602:i32)
            n460 = local read "从板个数"() -> (w617:dbl)
            n461 = local read "快换"() -> (w608:bool)
            n462 = Less Or Equal?(x=w603, y=w602) -> (x <= y?=w599:bool)
            n463 = call "输入数据解析.vi"("单个参数补充"=w617, "从板号"=w612, "主板引用"=w611, "从板引用"=w610, "主板选项"=w605, "枚举"=w609, "快换"=w608) -> ("输出数组"=w616:dbl[][], "数组长度"=w615:dbl[], "循环次数"=w607:i32, "命令"=w614:u32, "名称"=w606:string[], "命令序号"=w613:u32[])  [unwired: 2 in, 1 out]
            n464 = case shown="\"主板\", 默认" w609 {
              tunnel: w604 -> [w619 w633]
              frame "主板", Default {
                n465 = case shown="6" w619 {
                  tunnel: [T9."项目信息" ("主从板") T9."一级故障阀值" ("主从板") T9."二级故障阀值" ("主从板") T9."三级故障阀值" ("主从板") T9."控制参数" ("主从板") T9."电池信息" ("主从板")] -> w618
                  frame 0, Default {
                    n466 = local write "1"(TRUE ("1")) -> ()
                  }
                  frame 1 {
                    n467 = local write "1 2"(TRUE ("1 2")) -> ()
                  }
                  frame 2 {
                    n468 = local write "1 3"(TRUE ("1 3")) -> ()
                  }
                  frame 3 {
                    n469 = local write "1 4"(TRUE ("1 4")) -> ()
                  }
                  frame 4, 5 {
                    n470 = local write "1 5"(TRUE ("1 5")) -> ()
                  }
                  frame 6 {
                    n471 = local write "1 11"(TRUE ("1 11")) -> ()
                  }
                }
                n472 = local write "主板2"(w618) -> ()
              }
              frame "从板" {
                n473 = case shown="1" w633 {
                  tunnel: [T20."从板信息" ("等级 2") T20."从板信息" ("等级 2") T20."一级故障阀值" ("等级 2") T20."二级故障阀值" ("等级 2") T20."三级故障阀值" ("等级 2") T20."快换参数" ("等级 2") T15."均衡参数" ("等级 2")] -> w632
                  frame 99, Default {
                    n474 = local write "1 6"(TRUE ("1 6")) -> ()
                  }
                  frame 0 {
                    n475 = local write "1 6"(TRUE ("1 6")) -> ()
                  }
                  frame 1 {
                    n476 = local write "1 7"(TRUE ("1 7")) -> ()
                  }
                  frame 2 {
                    n477 = local write "1 8"(TRUE ("1 8")) -> ()
                  }
                  frame 3 {
                    n478 = local write "1 9"(TRUE ("1 9")) -> ()
                  }
                  frame 4 {
                    n479 = local write "1 10"(TRUE ("1 10")) -> ()
                  }
                  frame 5 {
                    n480 = local write "1 12"(TRUE ("1 10")) -> ()
                  }
                }
                n481 = local write "等级 2"(w632) -> ()
              }
            }
            n482 = for {
              N: w607 -> [w650]
              tunnel: w616 -> [w660]
              tunnel: w615 -> [w659]
              tunnel: w614 -> [w658]
              tunnel: w613 -> [w656]
              tunnel: w612 -> [w657]
              tunnel: w606 -> [w653]
              tunnel: w599 -> [w648]
              i -> [w649]
              n483 = Index Array(array=w660, index (row)=w649) -> (element=w655:dbl[])  [unwired: 1 in]
              n484 = Index Array(array=w659, index=w649) -> (element=w654:dbl)
              n485 = Index Array(array=w653, index=w649) -> (element=w651:string)
              n486 = Index Array(array=w656, index=w649) -> (element=w652:u32)
              n487 = stacked-sequence {
                seq-local: [_ _ _ w683 _ _] -> [_ _ _ _ w692 _]
                tunnel: w655 -> [_ _ w671 _ _ _]
                tunnel: w654 -> [_ _ w670 _ _ _]
                tunnel: w658 -> [_ _ w665 _ _ _]
                tunnel: w657 -> [_ _ w668 _ _ _]
                tunnel: w652 -> [_ _ w666 _ _ _]
                tunnel: w651 -> [_ _ w664 _ w691 _]
                tunnel: w650 -> [_ _ _ _ _ w704]
                tunnel: w649 -> [_ _ _ _ _ w703]
                tunnel: w648 -> [_ _ _ _ _ w701]
                frame #0 {
                  w662 = FALSE ("流控帧")
                  w661 = TRUE ("流控帧 2")
                  n488 = call <vilib>:"Set Busy.vi"("disable click? (T)"=w662) -> ()  [unwired: 3 in, 8 out]
                  n489 = global write "EV05全局变量1.vi" "读取超时"(w662) -> ()
                  n490 = global write "EV05全局变量1.vi" "流控帧"(w662) -> ()
                  n491 = local write "消除"(w661) -> ()
                  n492 = local write "控制1"(w661) -> ()
                  n493 = global write "EV05全局变量1.vi" "流控帧 2"(w661) -> ()
                  n494 = local write "写?"(w661) -> ()
                }
                frame #1 {
                  n495 = Wait Until Next ms Multiple(millisecond multiple=u32 50 ("毫秒倍数")) -> ()  [unwired: 1 out]
                }
                frame #2 {
                  n496 = global write "全局 1.vi" "名称"(w664) -> ()
                  n497 = local write "命令序号"(w666) -> ()
                  n498 = local write "命令"(w665) -> ()
